vi "LIA_Host.vi"() -> ()   [LabVIEW 2009]
uses:
  <vilib>/userDefined/High Color/nirio_resource_hc.ctl
  <vilib>/LabVIEW Targets/FPGA/cRIO/shared/nicrio_ModuleControls/nicrio_cRIO-9233_DataRatesRing.ctl
  <vilib>/rvi/interface/nirviOpenFPGA/nirviOpenFPGA.xnode
  FPGA Bitfiles/LIA.lvproj_FPGA Target_LIA_FPGA.vi.lvbitx
  LIA_FPGA.vi
  <vilib>/FPGAPlugInAG/cRIO-9104/nirviIntfOpen_cRIO-9104.vi
  <vilib>/rvi/interface/nirviMethod/nirviMethod.xnode
  <vilib>/rvi/ClientSDK/nirviWhatTheDeviceIsDoing.ctl
  <vilib>/rvi/interface/common/niFpgaNodeNameForErrorReporting.ctl
  <vilib>/rvi/errors/niLvFpgaWhatHappensToTopLevelVI.ctl
  <vilib>/Utility/error.llb/Merge Errors.vi
  <vilib>/LabVIEW Targets/FPGA/Rio/nirio_HostInterface/nirio_CleanUpAfterDownload.vi
  <vilib>/LabVIEW Targets/FPGA/Rio/nirio_HostInterface/nirio_ConfigureBitstreamVersion.vi
  <vilib>/LabVIEW Targets/FPGA/Rio/nirio_HostInterface/nirio_ConfigureRegisterAddresses.vi
  <vilib>/LabVIEW Targets/FPGA/Rio/nirio_HostInterface/nirio_PrepareForDownload.vi
  <vilib>/rvi/errors/niLvFpgaErrorClusterFromErrorCode.vi
  <vilib>/rvi/errors/nirviReportUnexpectedCaseInternalError.vi
  <vilib>/rvi/errors/nirviReportUnexpectedCaseInternalError (String).vi
  <vilib>/rvi/errors/nirviReportUnexpectedCaseInternalError (U32).vi
  <vilib>/RVI Host/nirviSupport.llb/nirviErrorClusterFromErrorCode.vi
  <vilib>/LabVIEW Targets/FPGA/Rio/nirio_HostInterface/nirio_ReadBig.vi
  <vilib>/LabVIEW Targets/FPGA/Rio/nirio_HostInterface/nirio_IsItOKToDownload.vi
  <vilib>/LabVIEW Targets/FPGA/Rio/nirio_HostInterface/nirio_Download.vi
  <vilib>/LabVIEW Targets/FPGA/Rio/nirio_HostInterface/nirio_DMAStopAll.vi
  <vilib>/LabVIEW Targets/FPGA/Rio/nirio_HostInterface/nirio_DisableInterrupts.vi
  <vilib>/Utility/error.llb/Error Cluster From Error Code.vi
  <vilib>/LabVIEW Targets/FPGA/Rio/nirio_HostInterface/nirio_Reset.vi
  <vilib>/rvi/errors/niLvFpgaReportInternalErrorWithAdditionalInfo.vi
  <vilib>/LabVIEW Targets/FPGA/Rio/nirio_HostInterface/nirio_DMAReconfigureDriver.vi
  <vilib>/LabVIEW Targets/FPGA/Rio/nirio_HostInterface/nirio_EnableInterrupts.vi
  <vilib>/LabVIEW Targets/FPGA/Rio/nirio_HostInterface/nirio_GetCompilationResults.vi
  <vilib>/rvi/FIFO/Fifo_Types/Fifo_DMA_Config.ctl
  <vilib>/rvi/DataTransferAndStorage/Container/Common/niFpgaDataTypeControl.ctl
  <vilib>/rvi/ClientSDK/Core/ModuleGeneration/CommunicationInterfaceUtility/niFpgaDmaChannelImplementation.ctl
  <vilib>/rvi/errors/niLvFpgaAdjustHostInterfaceError.vi
  <vilib>/rvi/interface/nirviReadWriteControl/nirviReadWriteControl.xnode
  <vilib>/LabVIEW Targets/FPGA/Rio/nirio_HostInterface/nirio_DMAConfigure.vi
  <vilib>/LabVIEW Targets/FPGA/Rio/nirio_HostInterface/nirio_WaitOnIRQ.vi
  <vilib>/rvi/interface/nirviCloseFPGA/nirviCloseFPGA.xnode
  <vilib>/FPGAPlugInAG/cRIO-9104/nirviIntfClose_cRIO-9104.vi
  NiRioSrv.dll
panel:
  out "Locked?":bool
  out "Locked Frequency [Hz]":dbl
  out "Phase [degree]":dbl
  out "Amplitude [V]":dbl
  in  "Data Rate":T1=2 items=["50.000 kS/s (NI 9233)"=2, "33.333 kS/s (NI 9233)"=3, "25.000 kS/s (NI 9233)"=34, "16.667 kS/s (NI 9233)"=35, "12.500 kS/s (NI 9233)"=36, "10.000 kS/s (NI 9233)"=37, "  8.333 kS/s (NI 9233)"=38, "  7.143 kS/s (NI 9233)"=39, "  6.250 kS/s (NI 9233)"=40, "  5.556 kS/s (NI 9233)"=41, "  5.000 kS/s (NI 9233)"=42, "  4.545 kS/s (NI 9233)"=43, "  4.167 kS/s (NI 9233)"=44, "  3.846 kS/s (NI 9233)"=45, "  3.571 kS/s (NI 9233)"=46, "  3.333 kS/s (NI 9233)"=47, "  3.125 kS/s (NI 9233)"=48, "  2.941 kS/s (NI 9233)"=49, "  2.778 kS/s (NI 9233)"=50, "  2.632 kS/s (NI 9233)"=51, "  2.500 kS/s (NI 9233)"=52, "  2.381 kS/s (NI 9233)"=53, "  2.273 kS/s (NI 9233)"=54, "  2.174 kS/s (NI 9233)"=55, "  2.083 kS/s (NI 9233)"=56, "  2.000 kS/s (NI 9233)"=57]
  out "Waveform Graph":sgl[][](graph)
  in  "stop":bool
  out "channel Q":dbl
  out "channel I":dbl
  in  "Nominal Freqency [Hz]":dbl=1000.0 format="%#.8g"
  in  "Filter Rolloff":enum16{"20 dB", "40 dB", "60 dB", "80 dB"}(ring)
  in  "Time Constant [s]":dbl=1.0 min=0.0 format="%.2f"
  in  "Resource Name":T2
  out "calib":cluster{"LSB Weight":u32, "Offset":i32}
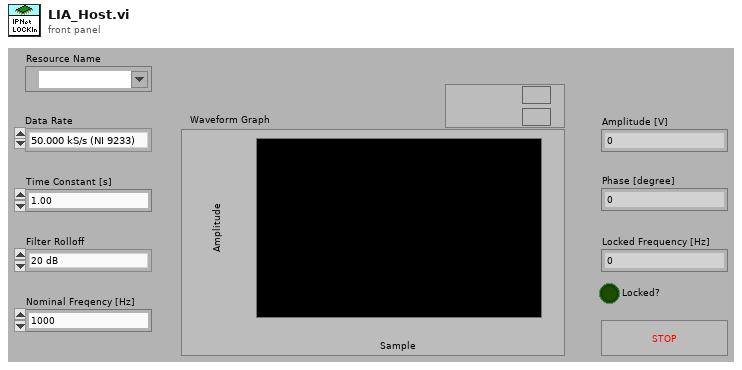
[diagram p1: front panel]
types:
  T1 = typedef "nicrio_cRIO-9233_DataRatesRing.ctl" = u8
  T2 = typedef "nirio_resource_hc.ctl" = tag
  T3 = typedef "niFpgaNodeNameForErrorReporting.ctl" = enum16{"Open FPGA VI Reference", "Read/Write Control", "Invoke Method: Abort", "Invoke Method: Acknowledge IRQ", "Invoke Method: Download", "Invoke Method: FIFO.Configure", "Invoke Method: FIFO.Read", "Invoke Method: FIFO.Start", "Invoke Method: FIFO.Stop", "Invoke Method: FIFO.Write", "Invoke Method: Reset", "Invoke Method: Run", "Invoke Method: Wait on IRQ", "Close FPGA VI Reference"}
  T4 = typedef "niLvFpgaWhatHappensToTopLevelVI.ctl" = enum16{"top level VI scripted behind XNode", "top level VI inlined behind XNode"}
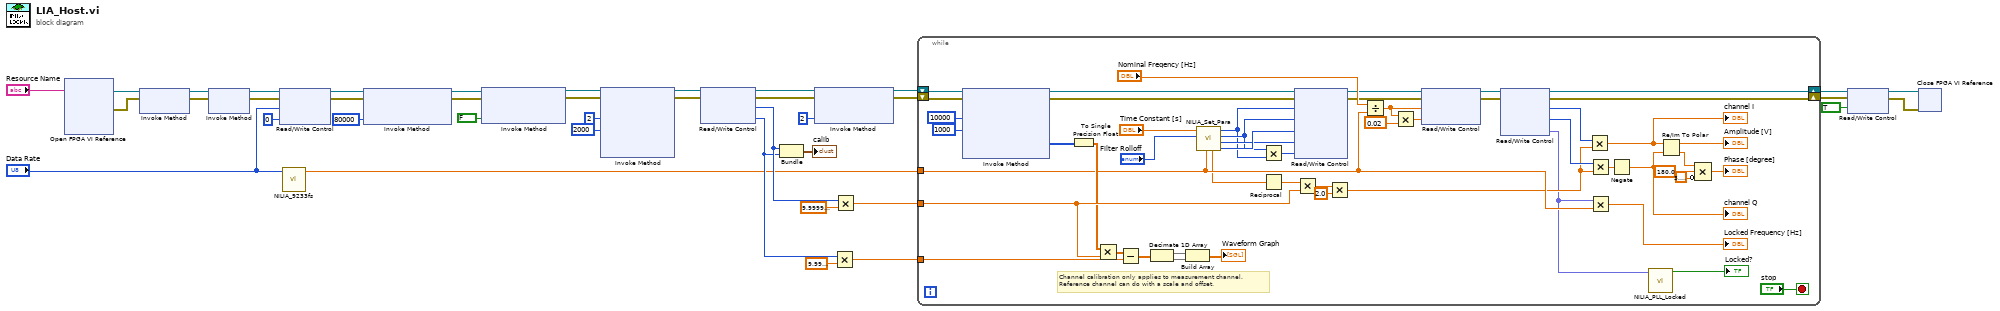
[diagram p0: block diagram]
diagram:
  n1 = xnode "Open FPGA VI Reference"("resource name"="Resource Name") -> ("FPGA VI Reference Out"=w39:refnum<k20>, "error out"=w38:errorcluster)  [unwired: 1 in]
  n2 = xnode "Invoke Method"("FPGA VI Reference In"=w39, "error in"=w38) -> ("FPGA VI Reference Out"=w37:refnum<k20>, "error out"=w36:errorcluster)
  n3 = xnode "Invoke Method"("FPGA VI Reference In"=w37, "error in"=w36) -> ("FPGA VI Reference Out"=w7:refnum<k20>, "error out"=w6:errorcluster)
  n4 = xnode "Read/Write Control"("FPGA VI Reference In"=w7, "error in"=w6, "Data Rate"="Data Rate", "channel"=i16 0) -> ("FPGA VI Reference Out"=w5:refnum<k20>, "error out"=w4:errorcluster)
  n5 = call "NILIA_9233fs.vi"("Data Rate"="Data Rate") -> ("fs"=w2:dbl)  [unwired: 10 in]
  n6 = xnode "Invoke Method"("FPGA VI Reference In"=w5, "error in"=w4, "Depth"=u32 80000) -> ("FPGA VI Reference Out"=w23:refnum<k20>, "error out"=w22:errorcluster)
  n7 = xnode "Invoke Method"("FPGA VI Reference In"=w23, "error in"=w22, "Wait Until Done (F)"=FALSE) -> ("FPGA VI Reference Out"=w31:refnum<k20>, "error out"=w30:errorcluster)
  n8 = xnode "Invoke Method"("FPGA VI Reference In"=w31, "error in"=w30, "IRQ Number(s)"=2, "Timeout (ms)"=2000) -> ("FPGA VI Reference Out"=w29:refnum<k20>, "error out"=w28:errorcluster)  [unwired: 2 out]
  n9 = xnode "Read/Write Control"("FPGA VI Reference In"=w29, "error in"=w28) -> ("FPGA VI Reference Out"=w32:refnum<k20>, "error out"=w25:errorcluster, "LSB Weight"=w19:u32, "Offset"=w9:i32)
  n10 = Bundle("LSB Weight"=w19, "Offset"=w9) -> (→"calib":cluster{"LSB Weight":u32, "Offset":i32})  [unwired: 1 in]
  n11 = xnode "Invoke Method"("FPGA VI Reference In"=w32, "error in"=w25, "IRQ Number(s)"=2) -> ("FPGA VI Reference Out"=w21:refnum<k20>, "error out"=w20:errorcluster)
  n12 = Multiply(x=w9, y=sgl 1e-09) -> (x*y=w8:sgl)
  n13 = Multiply(x=w19, y=sgl 1e-12) -> (x*y=w17:sgl)
  n14 = while {
    shift-right: [w88] -> w16
    shift-left: w21 -> [w82]
    shift-right: [w87] -> w15
    shift-left: w20 -> [w81]
    tunnel: w17 -> [w77]
    tunnel: w8 -> [w78]
    tunnel: w2 -> [w71]
    stop <- "stop" stop-if-true
    # "Channel calibration only applies to measurement channel.\nReference channel can do with a scale and offset."
    n15 = xnode "Invoke Method"("FPGA VI Reference In"=w82, "error in"=w81, "Number of Elements"=u32 10000, "Timeout (ms)"=1000) -> ("FPGA VI Reference Out"=w80:refnum<k20>, "error out"=w79:errorcluster, "Data"=w40:i32[])  [unwired: 1 out]
    n16 = To Single Precision Float(number=w40) -> (single precision float=w76:sgl[])
    n17 = Multiply(x=w76, y=w77) -> (x*y=w83:sgl[])
    n18 = Subtract(x=w83, y=w78) -> (x-y=w73:sgl[])
    n19 = Decimate 1D Array(w73) -> (w74:sgl[], w75:sgl[])
    n20 = Build Array(w74, w75) -> (→"Waveform Graph":sgl[][])
    n21 = call "NILIA_Set_Para.vi"("fs"=w71, "rolloff"="Filter Rolloff", "TC [sec]"="Time Constant [s]") -> ("3rd stages"=w57:i32, "3rd decimation"=w56:i32, "2nd decimation"=w55:i32, "1st decimation"=w54:i32, "corr"=w51:dbl)  [unwired: 4 in]
    n22 = Multiply(x=w55, y=w54) -> (x*y=w58:i32)
    n23 = Reciprocal(x=w51) -> (1/x=w50:dbl)
    n24 = xnode "Read/Write Control"("FPGA VI Reference In"=w80, "error in"=w79, "dec1"=w54, "dec2"=w55, "stages"=w57, "decimation"=w56, "dec"=w58) -> ("FPGA VI Reference Out"=w61:refnum<k20>, "error out"=w62:errorcluster)
    n25 = Multiply(x=w50, y=w77) -> (x*y=w49:dbl)
    n26 = Multiply(x=w49, y=2.0) -> (x*y=w45:dbl)
    n27 = Divide(x="Nominal Freqency [Hz]", y=w71) -> (x/y=w43:dbl)
    n28 = Multiply(x=w43, y=0.02) -> (x*y=w59:dbl)
    n29 = xnode "Read/Write Control"("FPGA VI Reference In"=w61, "error in"=w62, "nominal freq"=w43, "K"=w59) -> ("FPGA VI Reference Out"=w53:refnum<k20>, "error out"=w52:errorcluster)
    n30 = xnode "Read/Write Control"("FPGA VI Reference In"=w53, "error in"=w52) -> ("FPGA VI Reference Out"=w88:refnum<k20>, "error out"=w87:errorcluster, "channelI"=w47:i64, "channelQ"=w46:i64, "f"=w42:fxp<+/-,32,0>)
    n31 = Multiply(x=w47, y=w45) -> (x*y=w70:dbl)
    "channel I" <- w70
    n32 = Multiply(x=w46, y=w45) -> (x*y=w44:dbl)
    n33 = Multiply(x=w42, y=w71) -> (x*y=→"Locked Frequency [Hz]":dbl)
    n34 = Negate(x=w44) -> (-x=w69:dbl)
    "channel Q" <- w69
    n35 = call "NILIA_PLL_Locked.vi"("f"=w42) -> ("locked"=→"Locked?":bool)  [unwired: 10 in]
    n36 = Re/Im To Polar(2:w69, 3:w70) -> (0:w67:dbl, 1:→"Amplitude [V]":dbl)
    n37 = Compound Arithmetic op=MULTIPLY(w67, 180.0 ("value"), invert 3.141592653589793) -> (→"Phase [degree]":dbl)
  }
  n38 = xnode "Read/Write Control"("FPGA VI Reference In"=w16, "error in"=w15, "stop"=TRUE) -> ("FPGA VI Reference Out"=w13:refnum<k20>, "error out"=w12:errorcluster)
  n39 = xnode "Close FPGA VI Reference"("FPGA VI Reference In"=w13, "error in"=w12) -> ()  [unwired: 1 out]
